vi "AMC Send Network Message.vi"(1 "Priority Message (F)":bool, 4 "Message Attributes":T1, 5 "Receiver Host":string, 6 "Acknowledge Message (F)":bool, 7 "Receiver Process":string, 8 "error in (no error)":errorcluster, 9 "Message Value":string, 10 "Message Name":string, 11 "Message Queue in":T2) -> (0 "error out":errorcluster, 3 "Message Queue out":T2)   [LabVIEW 2009]
doc: "This VI is used for compatibility with previous versions of the AMC library. Use the AMC VIs located in the <b>Data Communication >> Asynchronous Message Communication</b> palette."
uses:
  Message Queue.ctl
  Message.ctl
  <vilib>/NI/Tools/Keyed Array/KeyedArray.ctl
  AMC.lvlib
  <vilib>/NI/Tools/Keyed Array/Tools_KeyedArray.lvlib
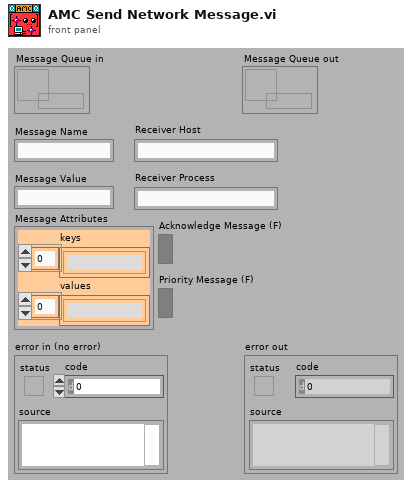
[diagram p1: front panel]
types:
  T1 = typedef "Tools_KeyedArray.lvlib/KeyedArray.ctl" = cluster{"keys":string[], "values":string[]}
  T2 = typedef "AMC.lvlib/Message Queue.ctl" = refnum<queue>
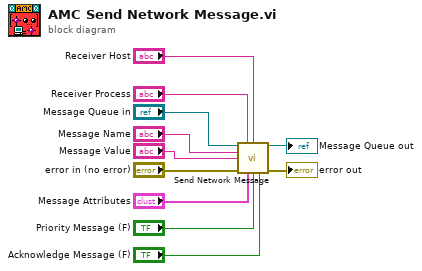
[diagram p0: block diagram]
diagram:
  n1 = call "Send Network Message.vi"("message queue in"="Message Queue in", "receiver process"="Receiver Process", "receiver host"="Receiver Host", "message name"="Message Name", "message value"="Message Value", "error in"="error in (no error)", "message attributes"="Message Attributes", "priority message (F)"="Priority Message (F)", "acknowledge message (F)"="Acknowledge Message (F)") -> ("message queue out"=→"Message Queue out":T2, "error out"=→"error out":errorcluster)  [unwired: 4 in, 1 out]
